vi "pixie collect data.vi"(8 "error in":errorcluster, 11 "Number of modules":T1) -> (0 "error out":errorcluster, 2 "mod2":u16[](array[numeric]), 3 "mode 0":u16[](array[numeric]), 4 "pixie runtime":dbl, 6 "Total time [s]":dbl)   [LabVIEW 2016]
doc: "uses the c code in the pixie 4 dll to get the raw data, runtime and total time. All of these are from the\npixie module"
uses:
  realtime data/pixie vis/controls/number of modules.ctl
  Drivers/Pixie4DLL.dll
panel:
  out "return type 2":u32
  out "return type":u32
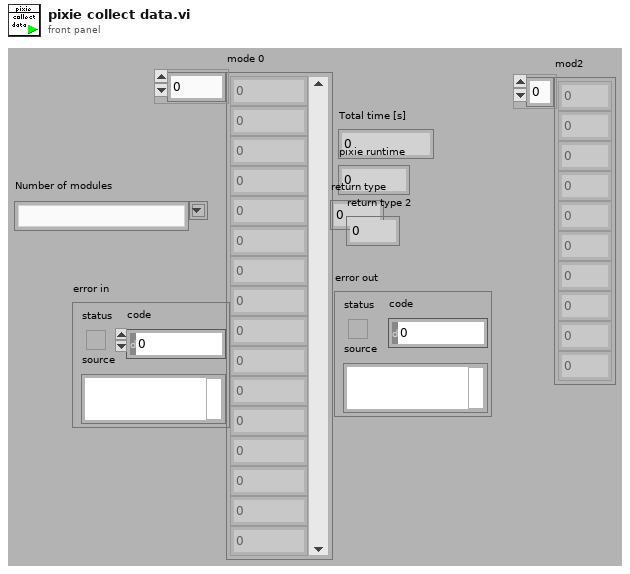
[diagram p1: front panel]
types:
  T1 = typedef "number of modules.ctl" = string
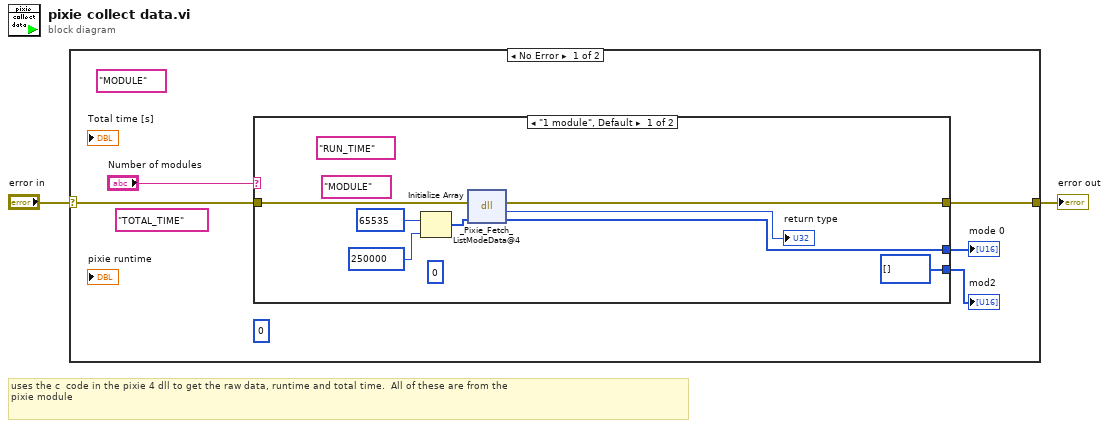
[diagram p0: block diagram]
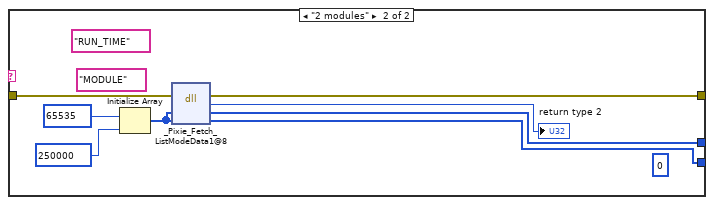
[diagram p2: hidden frame]
diagram:
  # "uses the c  code in the pixie 4 dll to get the raw data, runtime and total time.  All of these are from the\npixie module"
  n1 = case shown="No Error" "error in" {
    selector: "error in" -> [w7 w24]
    tunnel: [w6 w24] -> w2
    frame No Error {
      (unwired) 0
      (unwired) "MODULE"
      (unwired) "TOTAL_TIME"
      n2 = case shown="\"1 module\", Default" "Number of modules" {
        tunnel: w7 -> [w12 w21]
        tunnel: [w10 w19] -> w6
        tunnel: [w9 w18] -> w5
        tunnel: [u16[] [] ("buffer2") w16] -> w4
        frame "1 module", Default {
          (unwired) 0
          (unwired) "MODULE"
          (unwired) "RUN_TIME"
          n3 = Initialize Array(u16 65535 ("element"), u32 250000 ("dimension size")) -> (w15:u16[])
          n4 = dll-call lib="D:/Users/wymanm/Desktop/DAQuiri - 2017a/lois/Drivers/Pixie4DLL.dll" fn="_Pixie_Fetch_ListModeData@4"(error in=w12, "buffer1"=w15) -> (error out=w10:errorcluster, "return type"=→"return type":u32, "buffer1"=w9:u16[])  [unwired: 2 in, 1 out]
        }
        frame "2 modules" {
          (unwired) 0
          (unwired) "MODULE"
          (unwired) "RUN_TIME"
          n5 = Initialize Array(u16 65535 ("element"), u32 250000 ("dimension size")) -> (w17:u16[])
          n6 = dll-call lib="D:/Users/wymanm/Desktop/DAQuiri - 2017a/lois/Drivers/Pixie4DLL.dll" fn="_Pixie_Fetch_ListModeData1@8"(error in=w21, "buffer1"=w17, "buffer2"=w17) -> (error out=w19:errorcluster, "return type"=→"return type 2":u32, "buffer1"=w18:u16[], "buffer2"=w16:u16[])  [unwired: 2 in, 1 out]
        }
      }
      "mode 0" <- w5
      "mod2" <- w4
    }
    frame Error {
    }
  }
  "error out" <- w2
